vi "from string.vi"(8 "error in":errorcluster, 9 "data":string, 10 "version":string, 11 "Calculated Tags configuration in":refnum<class "Calculated Tags configuration.lvclass">) -> (0 "error out":errorcluster, 3 "Calculated Tags configuration out":refnum<class "Calculated Tags configuration.lvclass">)   [LabVIEW 2014, in "Calculated Tags configuration.lvclass"]
doc: "Provides an interface for loading a module configuration from a file or other serialized data source. It is recommended that all children of this class store data in two sets--data required for its own initialization, and any data required for parent initialization--and that each implementation uses the <b>Call Parent Method</b> primitive to de-serialize parent information. As a result, it is expected that every module configuration class calls <b>component configuration.lvclass:From String.vi</b>."
uses:
  Calculated Tags configuration.lvclass
  <vilib>/NI/Tag Bus Module Framework/module configuration/TBM module configuration.lvclass
  <vilib>/NI/Configuration Framework/serializable configuration/NISE_CEF_serializable configuration.lvclass
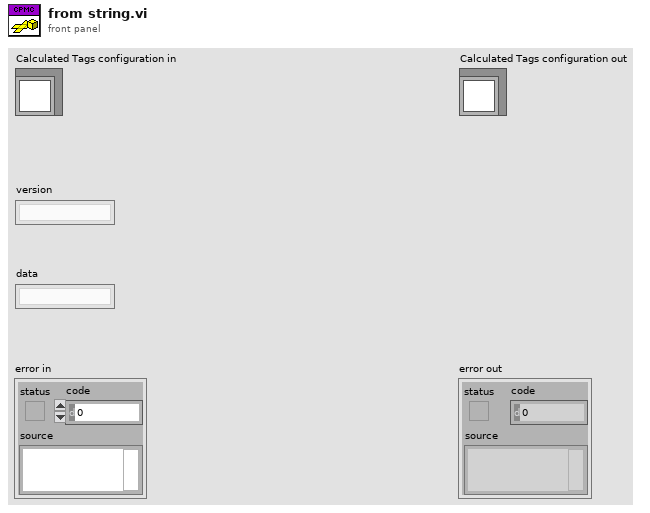
[diagram p1: front panel]
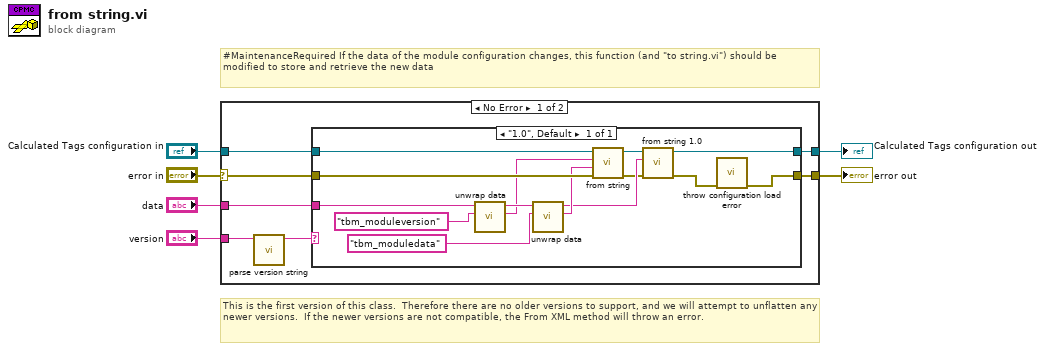
[diagram p0: block diagram]
diagram:
  # "#MaintenanceRequired If the data of the module configuration changes, this function (and \"to string.vi\") should be modified to store and retrieve the new data"
  # "This is the first version of this class.  Therefore there are no older versions to support, and we will attempt to unflatten any newer versions.  If the newer versions are not compatible, the From XML method will throw an error."
  n1 = case shown="No Error" "error in" {
    selector: "error in" -> [w7 w29]
    tunnel: "data" -> [w13 _]
    tunnel: "Calculated Tags configuration in" -> [w12 w28]
    tunnel: [w11 w28] -> w5
    tunnel: [w10 w29] -> w4
    tunnel: "version" -> [w9 _]
    frame No Error {
      n2 = call <vilib>:"parse version string.vi"("full version"=w9) -> ("major.minor version"=w8:string)  [unwired: 7 in, 3 out]
      n3 = case shown="\"1.0\", Default" w8 {
        tunnel: w13 -> [w24]
        tunnel: w7 -> [w23]
        tunnel: w12 -> [w27]
        tunnel: [w16] -> w11
        tunnel: [w26] -> w10
        frame "1.0", Default {
          n4 = call <vilib>:"unwrap data.vi"("identifier"="tbm_moduleversion" ("additional identifier"), "data to unwrap"=w24) -> ("unwrapped data"=w19:string, "remaining string"=w25:string)  [unwired: 8 in]
          n5 = call <vilib>:"unwrap data.vi"("identifier"="tbm_moduledata" ("additional identifier"), "data to unwrap"=w25) -> ("unwrapped data"=w21:string, "remaining string"=w18:string)  [unwired: 8 in]
          n6 = call-parent "from string.vi"("error in"=w23, "data"=w21, "version"=w19, "module configuration in"=w27) -> ("error out"=w15:errorcluster, "module configuration out"=w17:refnum<class "Calculated Tags configuration.lvclass">)  [unwired: 6 in]
          n7 = call "from string 1.0.vi"("error in (no error)"=w15, "data"=w18, "Calculated Tags configuration in"=w17) -> ("error out"=w14:errorcluster, "Calculated Tags configuration out"=w16:refnum<class "Calculated Tags configuration.lvclass">)  [unwired: 7 in]
          n8 = call <vilib>:"throw configuration load error.vi"("error in"=w14) -> ("error out"=w26:errorcluster)  [unwired: 10 in]
        }
      }
    }
    frame Error {
    }
  }
  "error out" <- w4
  "Calculated Tags configuration out" <- w5
